vi "Run.vi"(8 "error in (no error)":errorcluster, 11 "Power Meter GUI in":refnum<class "Power Meter GUI.lvclass">) -> (0 "error out":errorcluster, 1 "Parameters":cluster{"Name":string, "Value":string}[](array[cluster]), 2 "Canceled":bool, 3 "Power Meter GUI out":refnum<class "Power Meter GUI.lvclass">)   [LabVIEW 2020, in "Power Meter GUI.lvclass"]
doc: "This is the main test vi. It is here that the test is implemented."
uses:
  Power Meter GUI.lvclass
  Instruments/Instrument.lvclass/Instrument.ctl
  Instruments/Power Meter/Power Meter.lvclass
  C:/Sandbox/RF Bench/Source Code/WiSpry Test Framework/Instruments/Instrument.lvclass
  <instrlib>/Agilent U2000 Series/Public/Data/Low Level/Initiate (Continuous).vi
  <instrlib>/Agilent U2000 Series/Agilent U2000 Series.lvlib
  Instruments/Instrument.lvclass
panel:
  out "Array":refnum<visa-resource-name>[](array[refnum])
  in  "Continuous mode":bool
  in  "Stop Button":bool
  out "Power (dBm)":dbl[](array[numeric])
  in  "Power offset (dB)":dbl[](array[numeric])=[0.0, 0.0, 0.0, 0.0]
  out "String":string
  in  "Timeout (ms)":i32=500
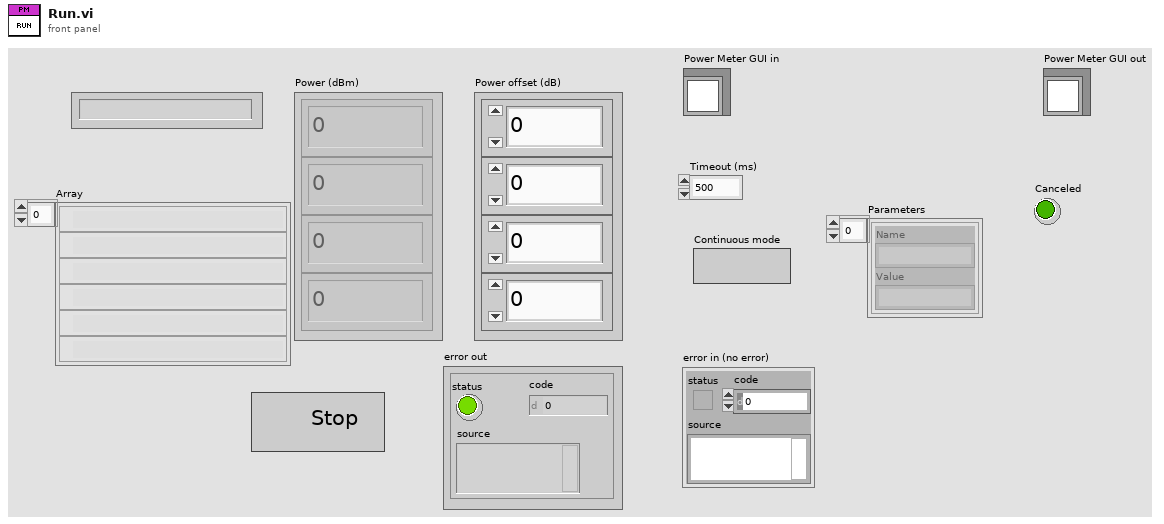
[diagram p1: front panel]
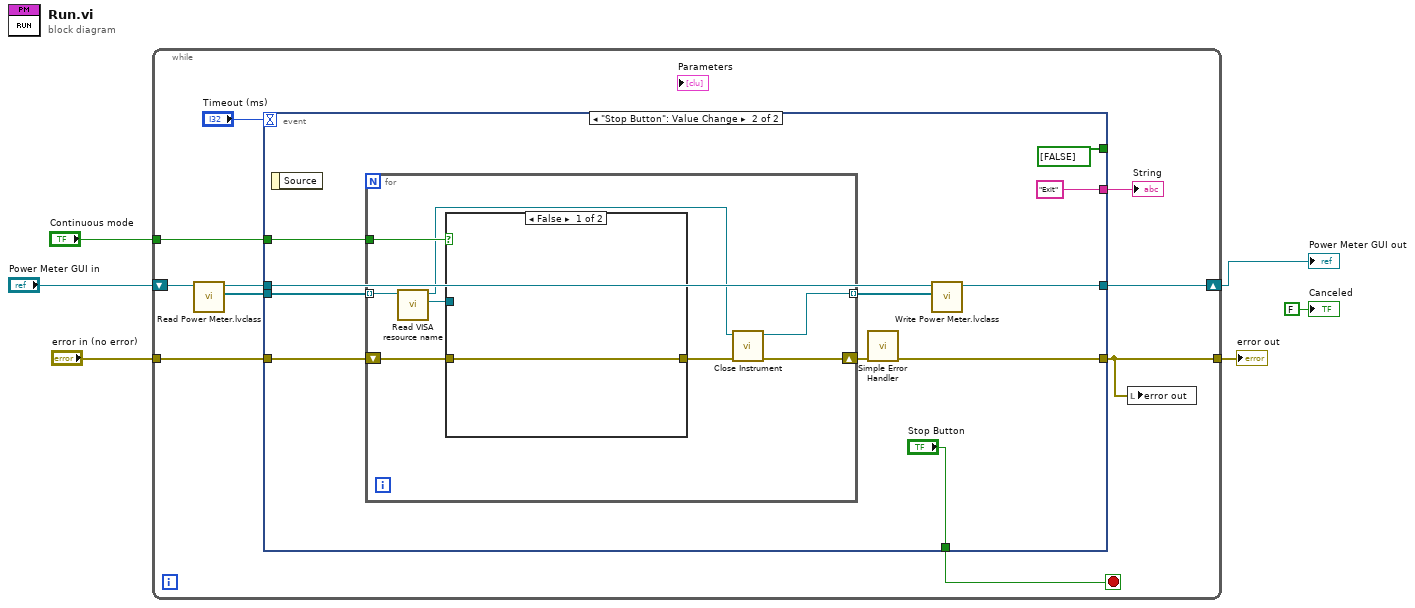
[diagram p0: block diagram]
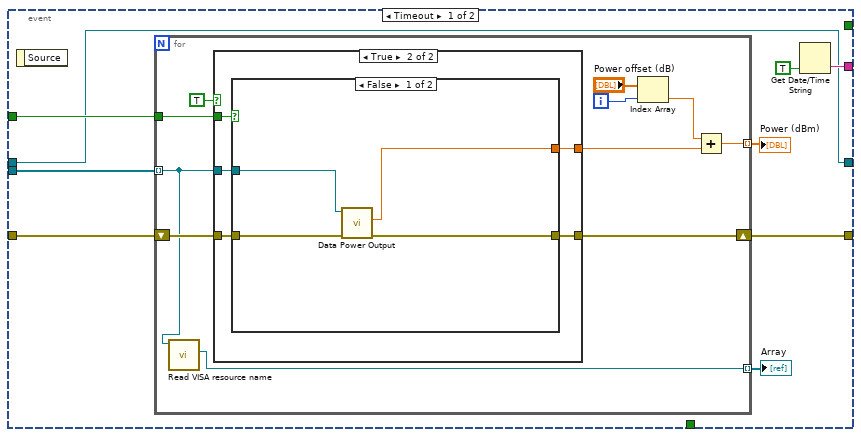
[diagram p2: hidden frame]
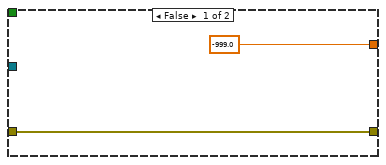
[diagram p3: hidden frame]
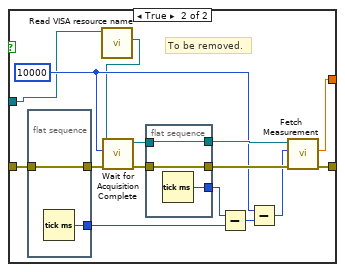
[diagram p4: hidden frame]
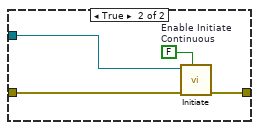
[diagram p5: hidden frame]
diagram:
  n1 = while {
    tunnel: "Continuous mode" -> [w11]
    tunnel: "error in (no error)" -> [w16]
    tunnel: [w15] -> w5
    shift-right: [w7] -> w2
    shift-left: "Power Meter GUI in" -> [w10]
    stop <- w14 stop-if-true
    n2 = call-dynamic "Read Power Meter.lvclass.vi"("Power Meter GUI in"=w10) -> ("Power Meters"=w9:refnum<class "Power Meter.lvclass">[], "Power Meter GUI out"=w8:refnum<class "Power Meter GUI.lvclass">)  [unwired: 9 in]
    n3 = event shown="[1] \"Stop Button\": Value Change" {
      selector: _ -> [_ _]
      dyn-events: _ -> [_ _]
      timeout: "Timeout (ms)" -> [_ _]
      tunnel: [w24 w74] -> w15
      tunnel: w16 -> [w25 w76]
      tunnel: [_ "Stop Button"] -> w14
      tunnel: [_ bool[] [FALSE]] -> _
      tunnel: [w23 "Exit" ("time string")] -> w13
      tunnel: w11 -> [w22 w73]
      tunnel: w9 -> [w19 w71]
      tunnel: w8 -> [w18 w69]
      tunnel: [w18 w68] -> w7
      event Timeout {
        n4 = event-data() -> ()  [unwired: 1 in, 1 out]
        n5 = for {
          tunnel: w22 -> [w34]
          shift-right: [w35] -> w24
          shift-left: w25 -> [w36]
          tunnel: [w29] -> w20 mode=indexing
          tunnel: w19 -> [w27] mode=indexing
          tunnel: [w26] -> w17 mode=indexing
          i -> [w32]
          n6 = call "Read VISA resource name.vi"("Instrument in"=w27) -> ("VISA resource name"=w26:refnum<visa-resource-name>)  [unwired: 9 in, 1 out]
          n7 = case shown="True" TRUE {
            tunnel: w36 -> [w38 w42]
            tunnel: [w38 w43] -> w35
            tunnel: w34 -> [_ w41]
            tunnel: [-999.0 ("Measurement") w40] -> w30
            tunnel: w27 -> [_ w39]
            frame False {
            }
            frame True {
              n8 = case shown="False" w41 {
                tunnel: [w47 w62] -> w40
                tunnel: [w45 w61] -> w43
                tunnel: w42 -> [w46 w60]
                tunnel: w39 -> [w44 w49]
                frame False {
                  n9 = call-dynamic "Data Power Output.vi"("error in (no error)"=w46, "Power Meter in"=w44) -> ("error out"=w45:errorcluster, "Power Out"=w47:dbl)  [unwired: 7 in, 1 out]
                }
                frame True {
                  w50 = u32 10000 ("Timeout (10000 ms)")
                  # "To be removed."
                  n10 = flat-sequence {
                    tunnel: [w67] -> w59
                    tunnel: w60 -> [w67]
                    tunnel: [w66] -> w53
                    frame #0 {
                      n11 = Tick Count (ms)() -> (millisecond timer value=w66:u32)
                    }
                  }
                  n12 = call "Read VISA resource name.vi"("Instrument in"=w49) -> ("VISA resource name"=w48:refnum<visa-resource-name>)  [unwired: 9 in, 1 out]
                  n13 = call <instrlib>:"Wait for Acquisition Complete.vi"("error in (no error)"=w59, "Maximum Time (10000 ms)"=w50, "VISA resource name"=w48) -> ("error out"=w57:errorcluster, "VISA resource name out"=w58:refnum<visa-resource-name>)  [unwired: 7 out]
                  n14 = flat-sequence {
                    tunnel: [w65] -> w56
                    tunnel: w58 -> [w65]
                    tunnel: [w64] -> w55
                    tunnel: w57 -> [w64]
                    tunnel: [w63] -> w54
                    frame #0 {
                      n15 = Tick Count (ms)() -> (millisecond timer value=w63:u32)
                    }
                  }
                  n16 = Subtract(x=w54, y=w53) -> (x-y=w52:u32)
                  n17 = Subtract(x=w50, y=w52) -> (x-y=w51:u32)
                  n18 = call <instrlib>:"Fetch Measurement.vi"("error in (no error)"=w55, "Timeout (10000 ms)"=w51, "VISA resource name"=w56) -> ("error out"=w61:errorcluster, "Measurement"=w62:dbl)  [unwired: 6 in, 1 out]
                }
              }
            }
          }
          n19 = Index Array(array="Power offset (dB)", index=w32) -> (element=w31:dbl)
          n20 = Add(x=w31, y=w30) -> (x+y=w29:dbl)
        }
        "Power (dBm)" <- w20
        "Array" <- w17
        n21 = Get Date/Time String(want seconds? (F)=TRUE) -> (time string=w23:string)  [unwired: 2 in, 1 out]
      }
      event "Stop Button": Value Change {
        n22 = event-data() -> ()  [unwired: 1 in, 1 out]
        n23 = for {
          tunnel: w73 -> [w85]
          shift-right: [w82] -> w75
          shift-left: w76 -> [w86]
          tunnel: w71 -> [w81] mode=indexing
          tunnel: [w84] -> w70 mode=indexing
          n24 = call "Read VISA resource name.vi"("Instrument in"=w81) -> ("VISA resource name"=w79:refnum<visa-resource-name>, "Instrument out"=w80:refnum<class "Power Meter.lvclass">)  [unwired: 9 in]
          n25 = case shown="False" w85 {
            tunnel: w86 -> [w87 w90]
            tunnel: w79 -> [_ w89]
            tunnel: [w87 w88] -> w83
            frame False {
            }
            frame True {
              w91 = FALSE  # Enable Initiate Continuous
              n26 = call-poly <instrlib>:"Initiate.vi"("Enable Initiate Continuous (T: Enable)"=w91, "error in (no error)"=w90, "VISA resource name"=w89) -> ("error out"=w88:errorcluster)  [unwired: 7 in, 1 out]
            }
          }
          n27 = call-dynamic "Close Instrument.vi"("error in (no error)"=w83, "Instrument in"=w80) -> ("error out"=w82:errorcluster, "Instrument out"=w84:refnum<class "Power Meter.lvclass">)  [unwired: 8 in]
        }
        n28 = call <vilib>:"Simple Error Handler.vi"("error in (no error)"=w75) -> ("error out"=w74:errorcluster)  [unwired: 1 in, 7 out]
        n29 = call-dynamic "Write Power Meter.lvclass.vi"("Power Meters"=w70, "Power Meter GUI in"=w69) -> ("Power Meter GUI out"=w68:refnum<class "Power Meter GUI.lvclass">)  [unwired: 9 in]
      }
    }
    "String" <- w13
    n30 = local write "error out"(w15) -> ()
  }
  "error out" <- w5
  "Power Meter GUI out" <- w2
  "Canceled" <- FALSE ("Cancled")
